vi "Max from Banana and Crit.vi"(8 "error in (no error)":errorcluster, 10 "Return Code":T1=enum."Skip All", 11 "Monkey in":refnum<class "Monkey.lvclass">) -> (0 "error out":errorcluster, 2 "Return Code":T1, 3 "Monkey out":refnum<class "Monkey.lvclass">)   [LabVIEW 2020, in "Monkey.lvlib" / "Monkey.lvclass"]
uses:
  Monkey.lvclass
  Run Utilities/TypeDefs/Return Code.ctl
  Monkey.lvclass/Monkey.ctl
  Run Utilities/Run Utilities.lvlib
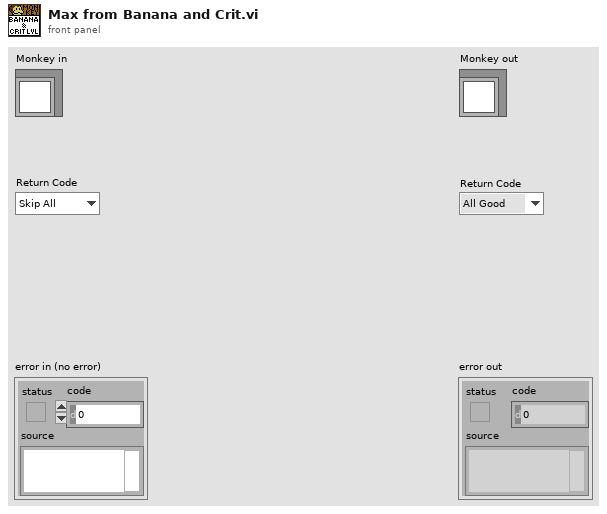
[diagram p1: front panel]
types:
  T1 = typedef "TALOS.lvlib/Run Utilities.lvlib/Return Code.ctl" = enum16{"All Good", "Retry", "Skip", "Skip All", "ABORT"}
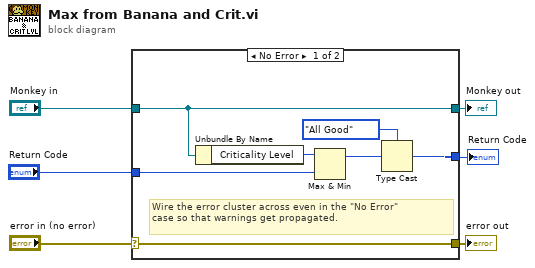
[diagram p0: block diagram]
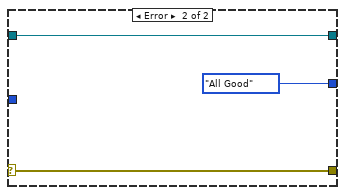
[diagram p2: hidden frame]
diagram:
  n1 = case shown="No Error" "error in (no error)" {
    selector: "error in (no error)" -> [w13 w16]
    tunnel: [w13 w16] -> w5
    tunnel: [w12 w15] -> w3
    tunnel: "Monkey in" -> [w12 w15]
    tunnel: "Return Code" -> [w11 _]
    tunnel: [w8 Return_Code."All Good" ("Return Code 2")] -> w1
    frame No Error {
      # "Wire the error cluster across even in the \"No Error\"\ncase so that warnings get propagated."
      n2 = Unbundle By Name(w12) -> ("Criticality Level"=w7:u8)
      n3 = Max & Min(x=w7, y=w11) -> (max(x,y)=w10:u16)  [unwired: 1 out]
      n4 = Type Cast(type=Return_Code."All Good" ("Return Code 2"), x=w10) -> (*(type *) &x=w8:T1)
    }
    frame Error {
    }
  }
  "error out" <- w5
  "Monkey out" <- w3
  "Return Code" <- w1
